vi "CRYUpdate After TS Write.vi"(8 "TS File path In":path, 11 "TS Edit Index In":i16) -> ()   [LabVIEW 2013]
uses:
  CRYProject Editor Global.vi
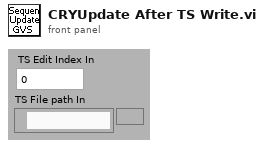
[diagram p1: front panel]
types:
  T1 = typedef "CRYTS.ctl" = cluster{"No.TS":u16, "TS File Path":path, "TS Name":string, "EditStepName":string, "Steps":T2[], "New State":bool, "Change State":bool, "Flattened CurveLib Data":string, "Document Data":string, "EditStepNo":u16, "Operator Start File":string, "Sequence Type":string, "Sequence Language":string}
  T2 = typedef "CRYStep.ctl" = cluster{"No.VI":i32, "Category":string, "StepName":string, "Seq setup flattened":string, "Comment":string, "Steps config.":bool[], "Jump config":i32[], "Start":dbl, "Increment":dbl, "Name":string, "Unit":string, "Y data":u16, "Y prefix":string, "Y dB ref":dbl, "Y unit":string, "Repeat State Array":cluster{"Start":dbl, "Increment":dbl, "Count":i32, "Num":i32}[]}
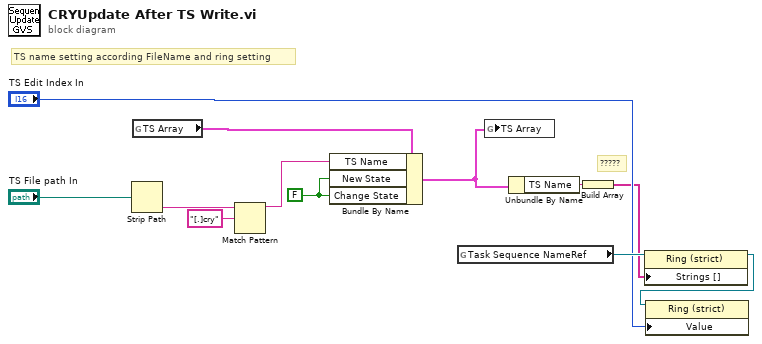
[diagram p0: block diagram]
diagram:
  w9 = FALSE ("Change Flag")
  # "?????"
  # "TS name setting according FileName and ring setting"
  n1 = Strip Path(path="TS File path In") -> (name=w12:string)  [unwired: 1 out]
  n2 = global read "CRYProject Editor Global.vi" "TS Array"() -> (w3:T1)
  n3 = Match Pattern(string=w12, regular expression="[.]cry") -> (before substring=w5:string)  [unwired: 4 out]
  n4 = Bundle By Name(cluster=w3, "TS Name"=w5, "New State"=w9, "Change State"=w9) -> (w2:T1)
  n5 = global read "CRYProject Editor Global.vi" "Task Sequence NameRef"() -> (w7:refnum<vi>)
  n6 = global write "CRYProject Editor Global.vi" "TS Array"(w2) -> ()
  n7 = Unbundle By Name(w2) -> ("TS Name"=w10:string)
  n8 = Build Array(w10) -> (w1:string[])
  n9 = property class="Ring (strict)"(reference=w7, "Strings []"=w1) -> (reference out=w6:refnum<vi>)  [unwired: 1 in, 1 out]
  n10 = property class="Ring (strict)"(reference=w6, "Value"="TS Edit Index In") -> ()  [unwired: 1 in, 2 out]
